vi "subvi_twice_bool_crossingA1.vi"(6 "Action":T1, 11 "Input Bool":bool=TRUE) -> (1 "First Half of Action Met?":bool, 3 "Action Met?":bool=TRUE)   [LabVIEW 2014]
doc: "Returns True if the Action condition has been met. \n\nThe last Input Bool is saved and compared to the Input Bool that came before it. If this boolean transition is the one required the First Half of Action is True. The last Input Bool is then compared to the current Input Bool and if this boolean transition is the one required AND the First Half of Action is True, then this function returns True."
uses:
  typedef_twice_bool_crossing.ctl
  typedef_boolcrossing.ctl
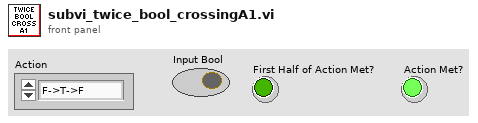
[diagram p1: front panel]
types:
  T1 = typedef "typedef_twice_bool_crossing.ctl" = enum16{"F->T->F", "T->F->T", "Initialise"}
  T2 = typedef "typedef_boolcrossing.ctl" = enum16{"Either", "True-False", "False-True", "Initialise"}
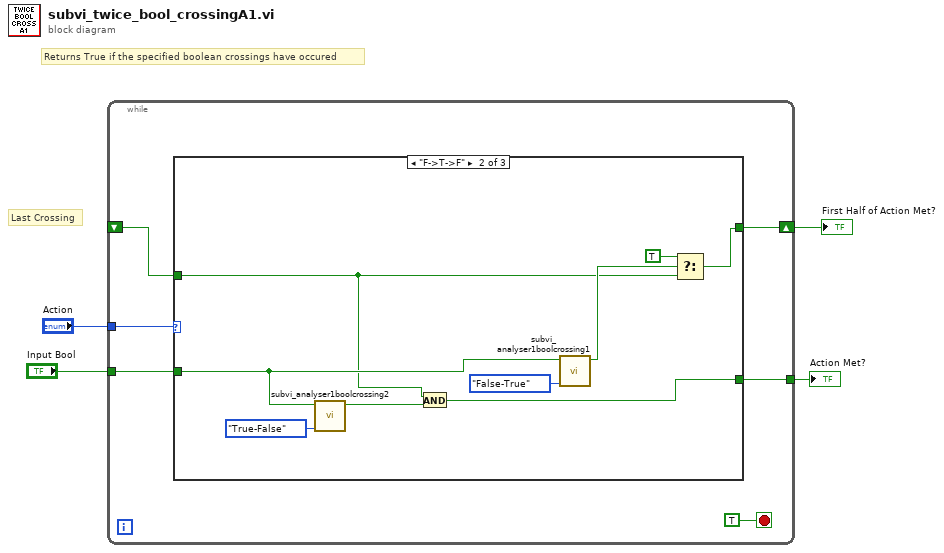
[diagram p0: block diagram]
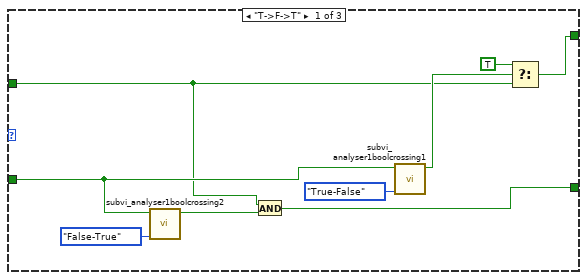
[diagram p2: hidden frame]
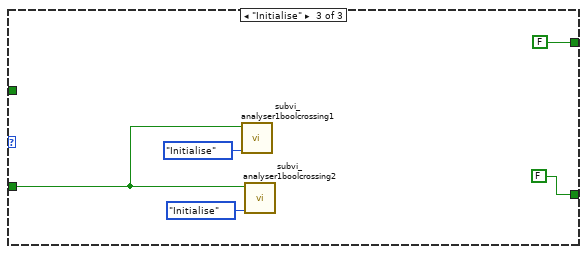
[diagram p3: hidden frame]
diagram:
  # "Last Crossing"
  # "Returns True if the specified boolean crossings have occured"
  n1 = while {
    tunnel: "Action" -> [w10]
    tunnel: "Input Bool" -> [w9]
    shift-right: [w7] -> w1
    shift-left: _ -> [w8]
    tunnel: [w6] -> w2
    stop <- TRUE stop-if-true
    n2 = case shown="\"F->T->F\"" w10 {
      tunnel: w9 -> [w19 w28 w31]
      tunnel: w8 -> [w11 w20 _]
      tunnel: [w13 w22 FALSE ("Crossed?")] -> w7
      tunnel: [w18 w27 FALSE ("Crossed?")] -> w6
      frame "T->F->T" {
        n3 = call "subvi_analyser1boolcrossing2.vi"("Action"=typedef_boolcrossing."False-True", "Input Bool"=w19) -> ("Crossed?"=w16:bool)  [unwired: 9 in]
        n4 = And(x=w11, y=w16) -> (x .and. y?=w18:bool)
        n5 = call "subvi_analyser1boolcrossing1.vi"("Action"=typedef_boolcrossing."True-False", "Input Bool"=w19) -> ("Crossed?"=w14:bool)  [unwired: 9 in]
        n6 = Select(t=TRUE, s=w14, f=w11) -> (s? t:f=w13:bool)
      }
      frame "F->T->F" {
        n7 = call "subvi_analyser1boolcrossing2.vi"("Action"=typedef_boolcrossing."True-False", "Input Bool"=w28) -> ("Crossed?"=w25:bool)  [unwired: 9 in]
        n8 = And(x=w20, y=w25) -> (x .and. y?=w27:bool)
        n9 = call "subvi_analyser1boolcrossing1.vi"("Action"=typedef_boolcrossing."False-True", "Input Bool"=w28) -> ("Crossed?"=w23:bool)  [unwired: 9 in]
        n10 = Select(t=TRUE, s=w23, f=w20) -> (s? t:f=w22:bool)
      }
      frame "Initialise" {
        n11 = call "subvi_analyser1boolcrossing1.vi"("Action"=typedef_boolcrossing."Initialise", "Input Bool"=w31) -> ()  [unwired: 9 in, 1 out]
        n12 = call "subvi_analyser1boolcrossing2.vi"("Action"=typedef_boolcrossing."Initialise", "Input Bool"=w31) -> ()  [unwired: 9 in, 1 out]
      }
    }
  }
  "Action Met?" <- w2
  "First Half of Action Met?" <- w1
